vi "Penta Panes Demo.vi"() -> ()   [LabVIEW 2023]
doc: "Overview: Demonstrates the use of PentaPanes Class using a mockup of a GUI window. \nRequirements: Labview 2023 or compatible. \nInstructions: \n1. Run \"Penta Panes Demo.vi\" \n2. Play around with the GUI to see how it behaves. :)"
uses:
  Penta Panes.lvlibp/PanesColors.ctl
  <vilib>/Utility/miscctls.llb/LVBoundsTypeDef.ctl
  Penta Panes.lvlibp/ResizeBehaviourCluster.ctl
  Penta Panes.lvlibp/BordersCluster.ctl
  Penta Panes.lvlibp/1abvi3w/vi.lib/Utility/miscctls.llb/LVBoundsTypeDef.ctl
  Penta Panes.lvlibp/PanePosition.ctl
  <vilib>/Platform/browser.llb/Open URL in Default Browser (string).vi
  Penta Panes.lvlibp/5PanesGUI.lvclass
  Penta Panes.lvlibp
panel:
  out "Logo":picture[](array[picture])=[bytes[15730], bytes[15730], bytes[15730], bytes[15730], bytes[15730], bytes[15730], bytes[15730], bytes[15730], bytes[15730], bytes[15730], bytes[15730], bytes[15730], bytes[15730], bytes[15730], bytes[15730], bytes[15730], bytes[15730], bytes[15730], bytes[15730], bytes[15730], bytes[15730], bytes[15730], bytes[15730], bytes[15730], bytes[15730], bytes[15730], bytes[15730], bytes[15730], bytes[15730], bytes[15730], bytes[15730], bytes[15730], bytes[15730], bytes[15730], bytes[15730], bytes[15730], bytes[15730], bytes[15730], bytes[15730], bytes[15730], bytes[15730], bytes[15730], bytes[15730], bytes[15730], bytes[15730], bytes[15730], bytes[15730], bytes[15730], bytes[15730], bytes[15730], bytes[15730], bytes[15730]]
  out "Icons Values":bool[](array[boolean])
  out "IconNames":string[](array[string])
  out "Icons":picture[](array[picture])=[bytes[7230], bytes[7230], bytes[7230], bytes[7230], bytes[7230], bytes[7230], bytes[7230], bytes[7230], bytes[7230], bytes[7230], bytes[7230], bytes[7230], bytes[7230], bytes[7230], bytes[7230], bytes[7230], bytes[7230], bytes[7230], bytes[7230], bytes[7230], bytes[7230], bytes[7230], bytes[7230], bytes[7230], bytes[7230], bytes[7230], bytes[7230], bytes[7230], bytes[7230], bytes[7230], bytes[7230], bytes[7230], bytes[7230], bytes[7230], bytes[7230], bytes[7230], bytes[7230], bytes[7230], bytes[7230], bytes[7230], bytes[7230], bytes[7230], bytes[7230], bytes[7230], bytes[7230], bytes[7230], bytes[7230], bytes[7230], bytes[7230], bytes[7230], bytes[7230], bytes[7230]]
  in  "Options Tree":string[](tree)=["About"]
  in  "Options Tab":T1(tab)
  in  "Developed By\nLEAP CODE\nLinking hardware \nwith software\n\nYoni Cohen":string="yoncoh@gmail.com"
  in  "Icon set by":string="https://icons8.com"
  out "about picture":picture
  in  "Graphs Layout":T2(ring)=enum."3 Line graphs"
  in  "Right Pane View":u16(ring) items=["First", "Second", "Third"]
  in  "Top Pane Size":i32=75 caption="Top"
  in  "Right Pane Size":i32=156 caption="Right" max=4000
  in  "Left Pane Size":i32=113 caption="Left"
  in  "Bottom Pane Size":i32=100 caption="Bottom"
  in  "Colors":T3
  out "FP Bounds":T4
  out "App Path":path=path "E:/Work/5PanesWindow/5PanesDemo.vi"
  out "Eventloop Error":errorcluster
  out "Init Error":errorcluster
  out "Intensity Graph 2":dbl[][](graph)
  out "XY Graph 3":cluster{dbl[], dbl[]}[](graph)
  out "XY Graph 2":cluster{dbl[], dbl[]}[](graph)
  out "XY Graph":cluster{dbl[], dbl[]}[](graph)
  out "Intensity Graph":dbl[][](graph)
  in  "Third pane Tab":enum32{"Page 1", "Page 2"}(tab)
  in  "First pane Tab":enum32{"Page 1", "Page 2"}(tab)
  in  "Second pane Tab":enum32{"Page 1", "Page 2"}(tab)
  in  "Listbox":i32(listbox)=-1
  # "Overview: A mockup of a GUI window demonstrating the use of \nthe \"PentaPanes\" Class\nRequirements: LabVIEW 2023 or \ncompatible \nInstructions: Run this VI and play \naround with the GUI. \nopen and close panes by pressing the white splitters."
  # "Panes"
  # "Sizes"
  # "Debug Pane"
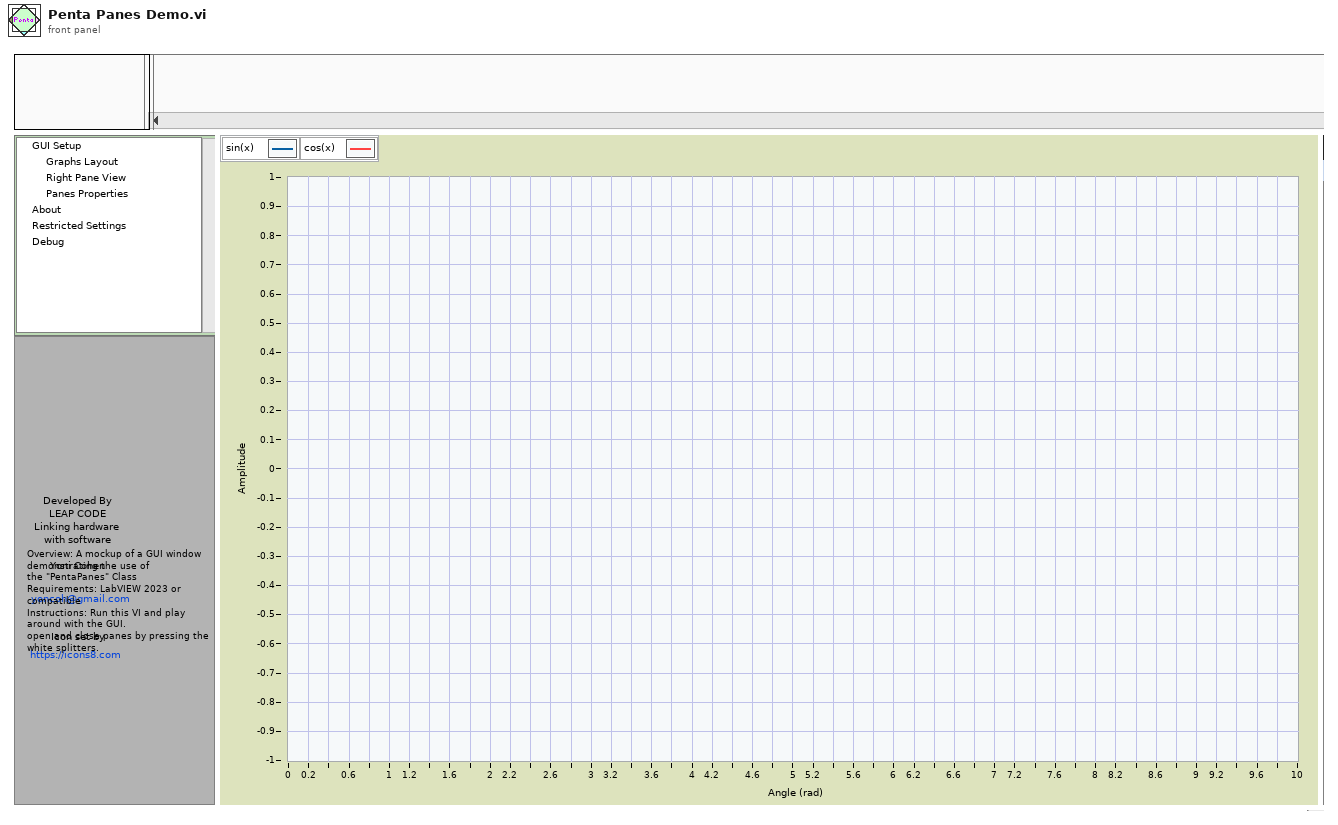
[diagram p1: front panel]
types:
  T1 = enum32{"About", "Graphs Layout", "Right Pane View", "Panes Colors", "Panes Properties", "Debug", "Restricted Settings"}
  T2 = enum16{"1 Line Graph", "1 Line + 2 Intensity", "3 Line graphs", "1 Intensity", "2 Intensity H", "2 Intensity V", "All"}
  T3 = typedef "Penta Panes.lvlibp/5PanesGUI.lvclass/PanesColors.ctl" = cluster{"Top Color":u32, "Left Color":u32, "Center Color":u32, "Right Color":u32, "Bottom Color":u32}
  T4 = typedef "LVBoundsTypeDef.ctl" = cluster{"Width":u32, "Height":u32}
  T5 = enum32{"Invalid", "Standard", "Closed", "Hidden", "Minimized", "Maximized"}
  T6 = enum16{"1 Line Graph", "1 Line + 2 Intensity", "3 Line graphs", "1 Intensity"}
  T7 = typedef "Penta Panes.lvlibp/5PanesGUI.lvclass/ResizeBehaviourCluster.ctl" = cluster{"Adjust":u16, "Borders":T8, "Borders in Percent?":bool, "Minimal":T9, "Invisible?":bool, "Force aspect ratio?":bool}
  T8 = typedef "Penta Panes.lvlibp/5PanesGUI.lvclass/BordersCluster.ctl" = cluster{"Left":i32, "Top":i32, "Right":i32, "Bottom":i32}
  T9 = typedef "Penta Panes.lvlibp/LVBoundsTypeDef.ctl" = cluster{"Width":u32, "Height":u32}
  T10 = typedef "LVRectTypeDef.ctl" = cluster{"Left":i16, "Top":i16, "Right":i16, "Bottom":i16}
  T11 = typedef "Penta Panes.lvlibp/5PanesGUI.lvclass/PanePosition.ctl" = u16
  T12 = typedef "LVPoint32TypeDef.ctl" = cluster{"Horizontal":i32, "Vertical":i32}
  T13 = typedef "LVRangeTypeDef.ctl" = cluster{"Minimum":dbl, "Maximum":dbl, "Increment":dbl, "Minor Increment":dbl, "Start":dbl}
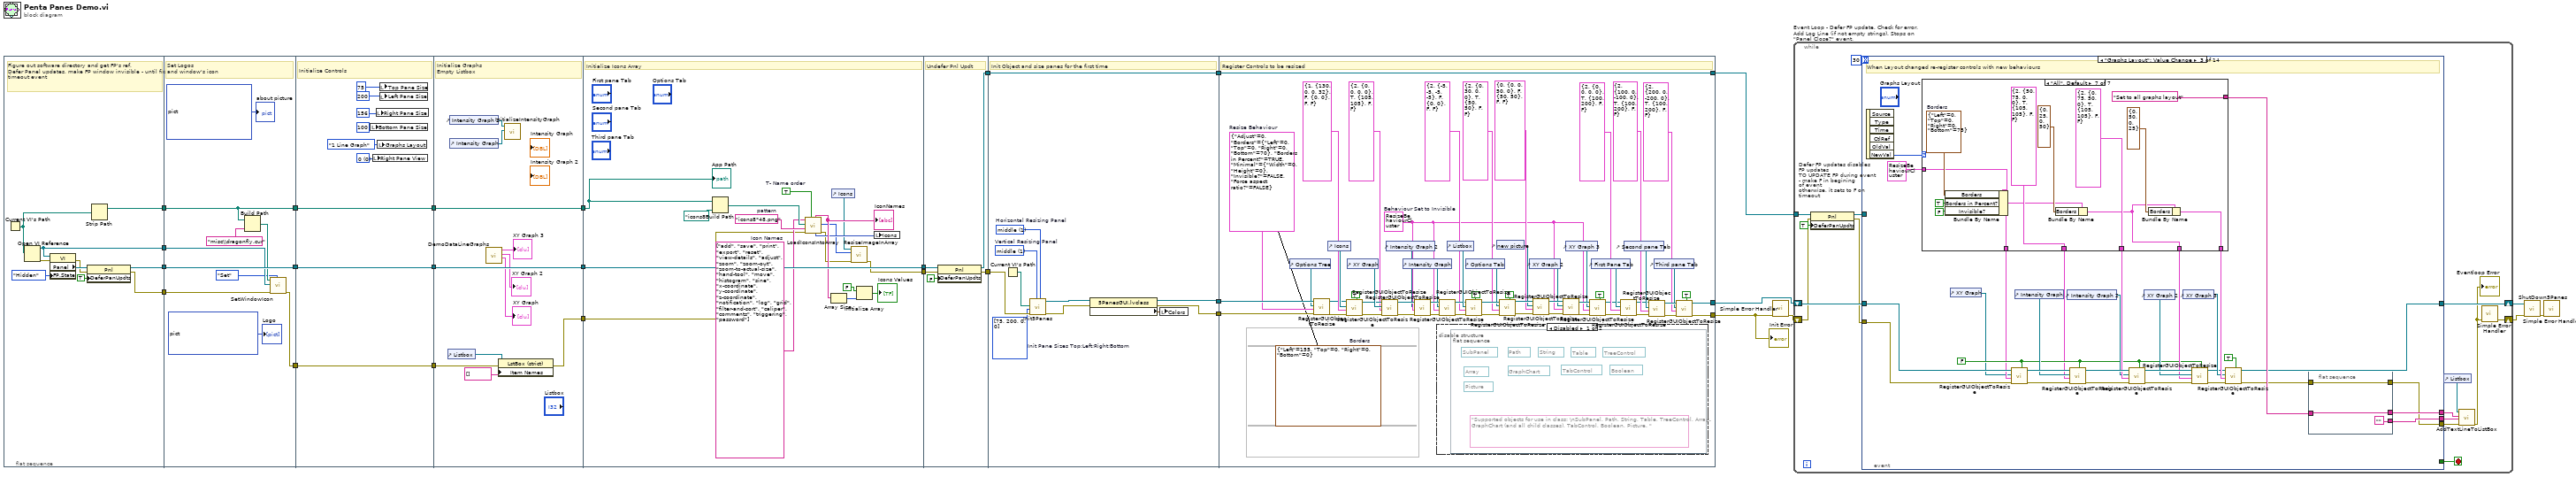
[diagram p0: block diagram]
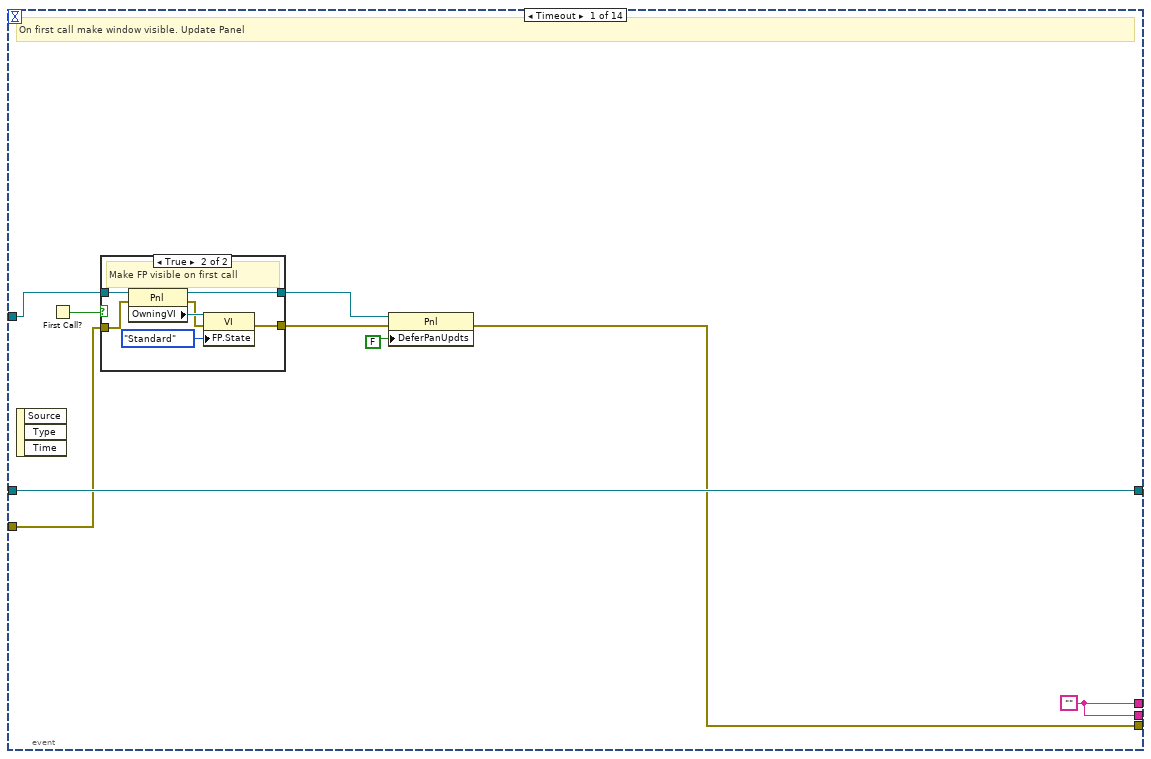
[diagram p3: hidden frame]
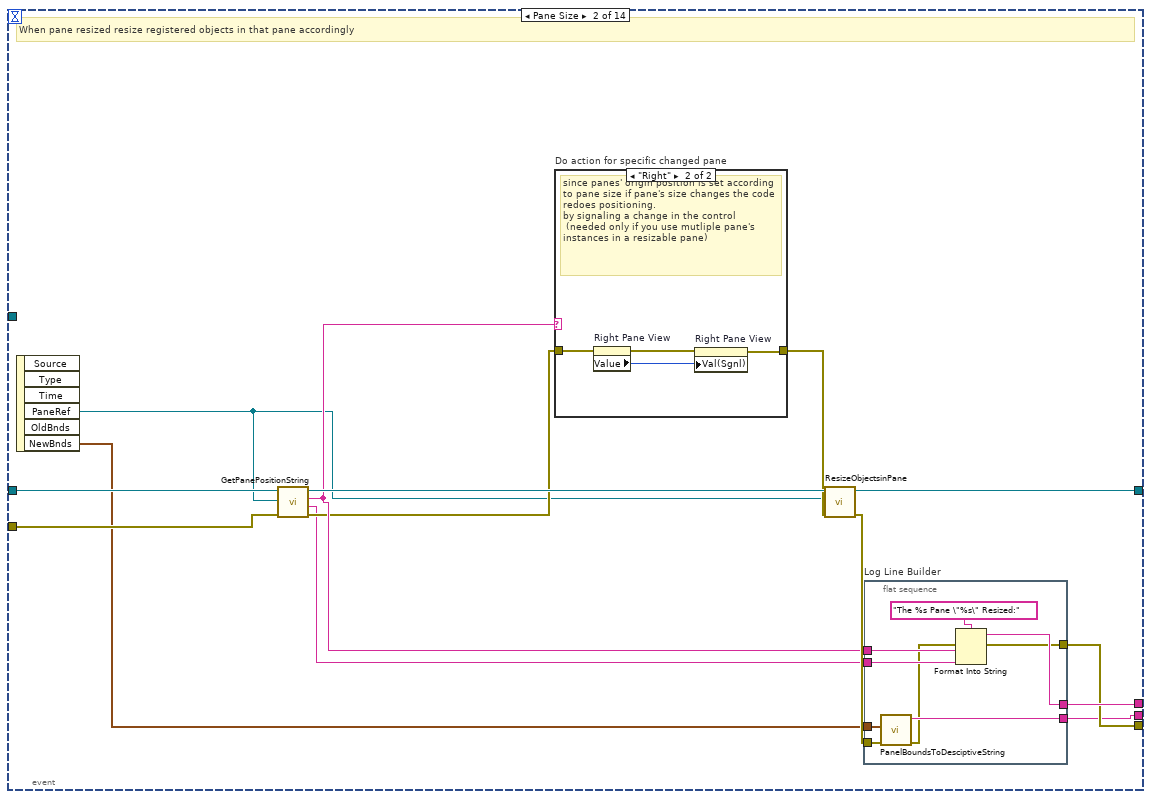
[diagram p5: hidden frame]
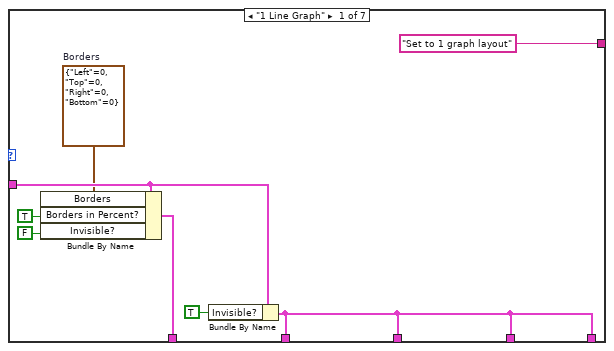
[diagram p7: hidden frame]
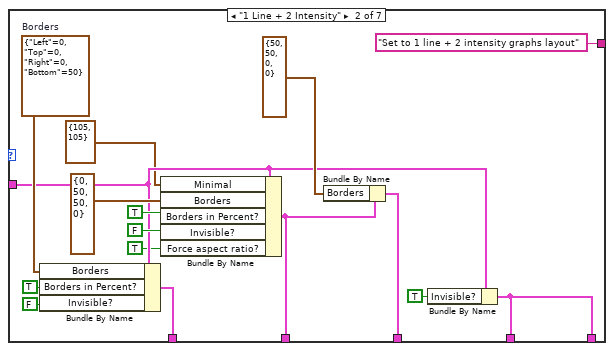
[diagram p8: hidden frame]
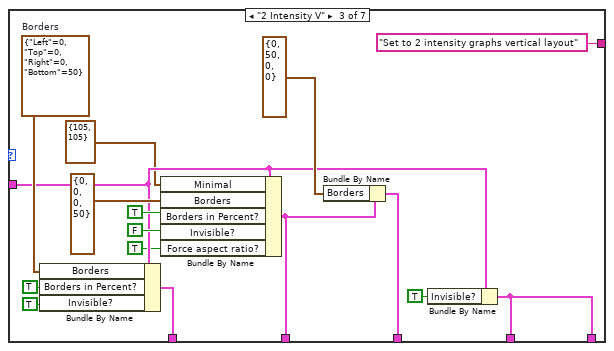
[diagram p9: hidden frame]
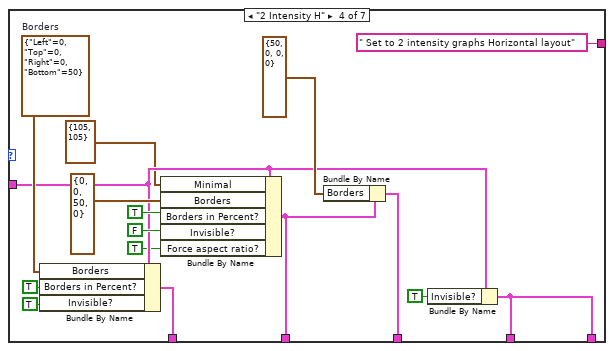
[diagram p10: hidden frame]
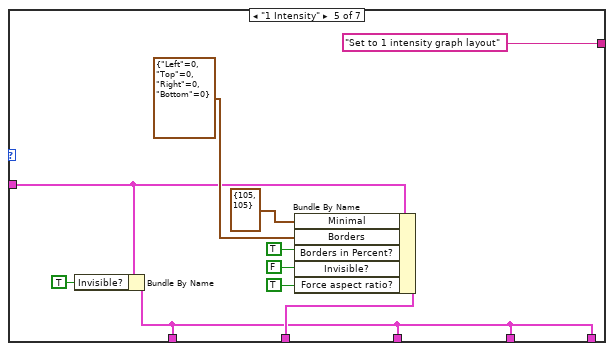
[diagram p11: hidden frame]
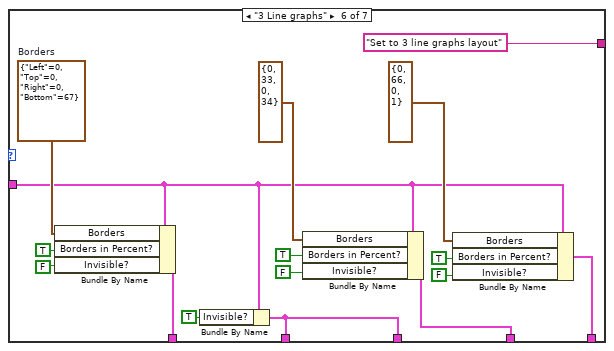
[diagram p12: hidden frame]
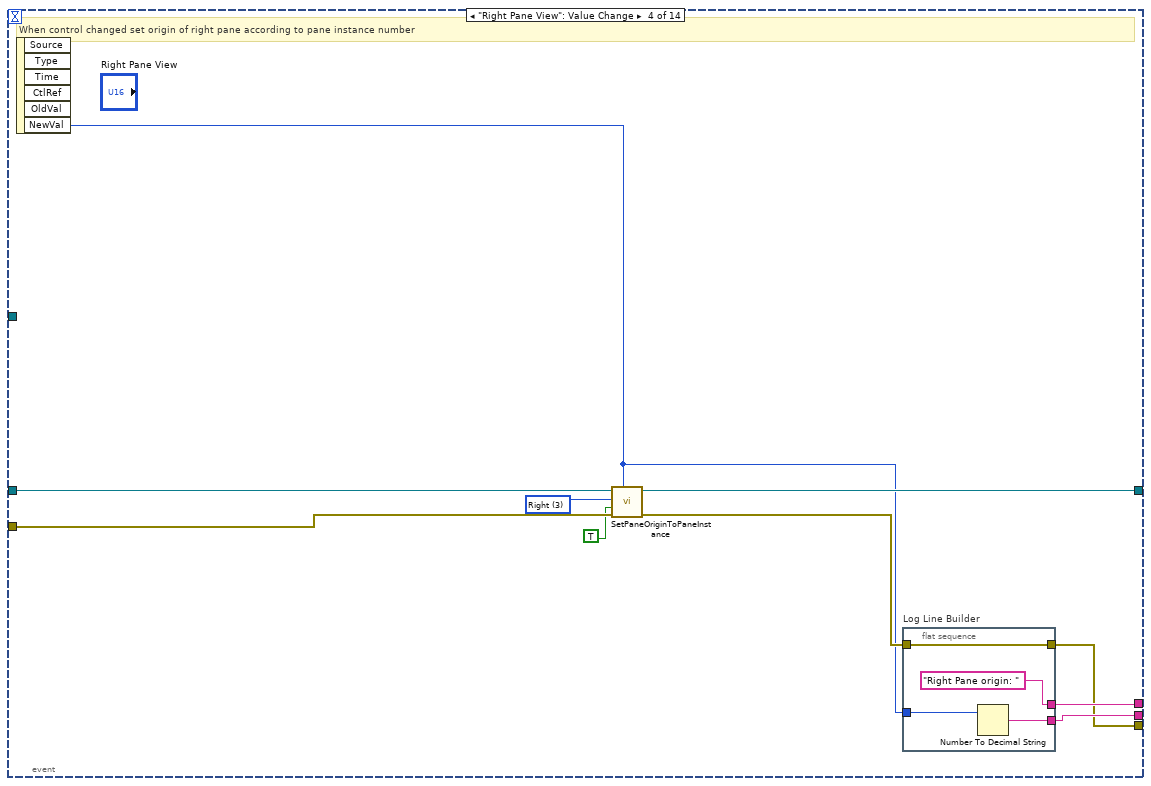
[diagram p13: hidden frame]
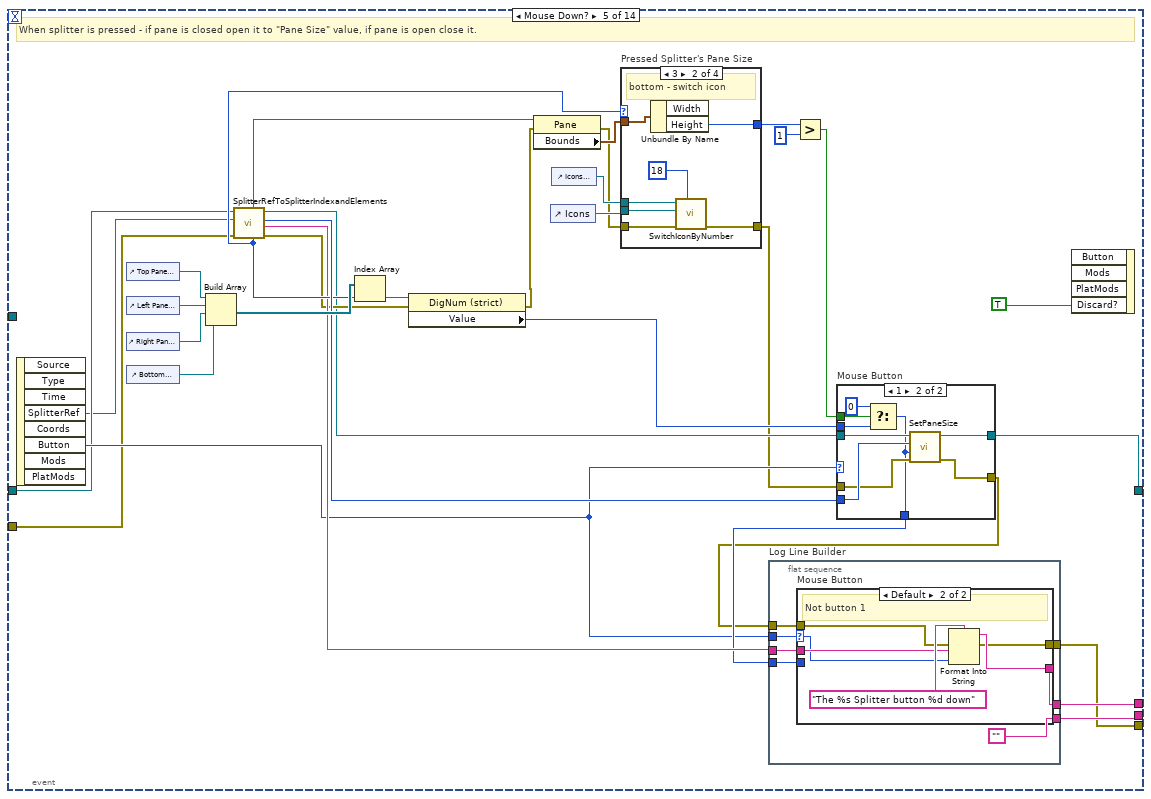
[diagram p14: hidden frame]
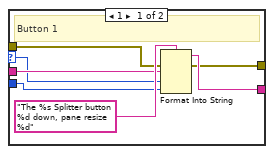
[diagram p15: hidden frame]
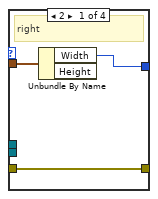
[diagram p16: hidden frame]
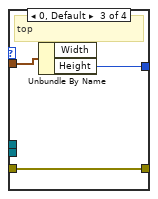
[diagram p17: hidden frame]
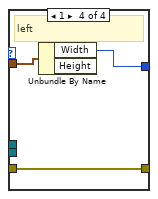
[diagram p18: hidden frame]
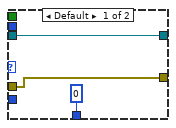
[diagram p19: hidden frame]
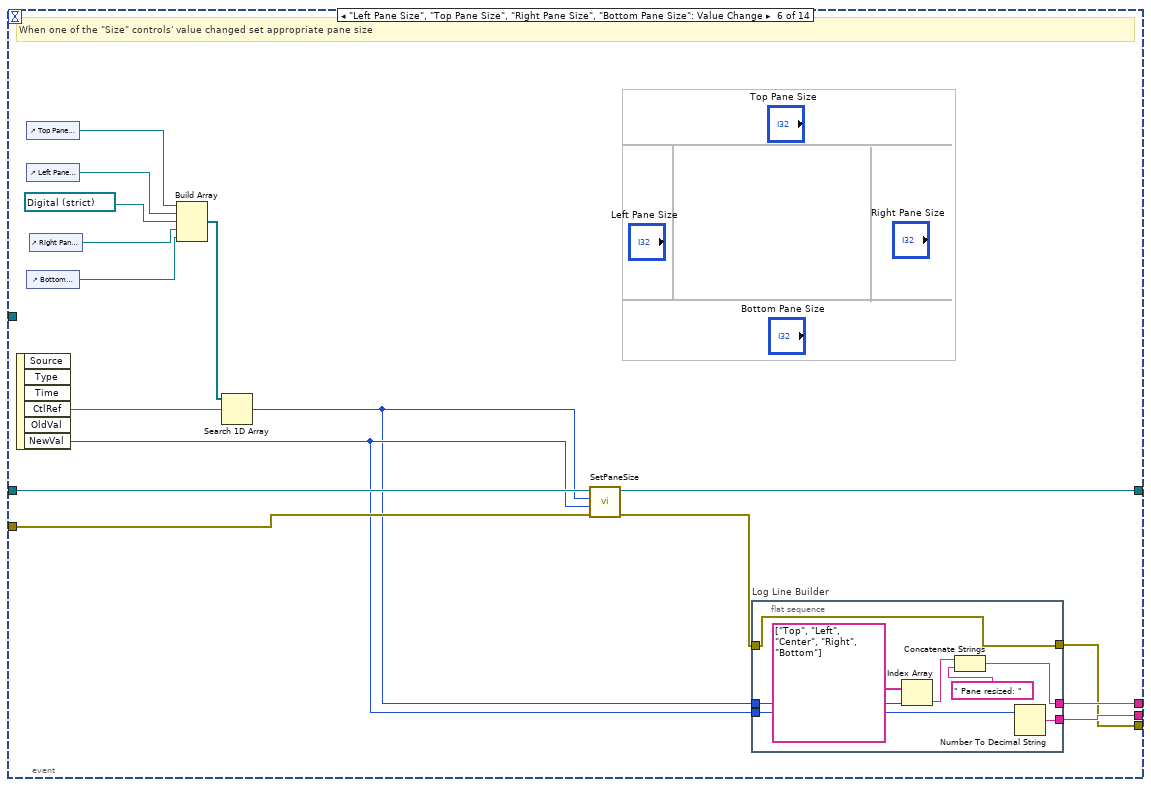
[diagram p20: hidden frame]
diagram:
  n1 = flat-sequence {
    tunnel: [w34] -> w12
    tunnel: [w32] -> w9
    tunnel: [w31] -> w8
    tunnel: [w29] -> w7
    tunnel: [w38] -> w13
    tunnel: w12 -> [w47]
    tunnel: [w47] -> w11
    tunnel: [w44] -> w10
    tunnel: w9 -> [w46]
    tunnel: w8 -> [w45]
    tunnel: w7 -> [w38]
    tunnel: w13 -> [w56]
    tunnel: [w56] -> w19
    tunnel: w11 -> [w55]
    tunnel: [w55] -> w17
    tunnel: [w48] -> w15
    tunnel: w10 -> [w48]
    tunnel: w19 -> [w67]
    tunnel: [w67] -> w18
    tunnel: w17 -> [w66]
    tunnel: [w66] -> w16
    tunnel: w15 -> [w59]
    tunnel: [w58] -> w14
    tunnel: [w84] -> w24
    tunnel: w18 -> [w74]
    tunnel: w16 -> [w84]
    tunnel: [w70] -> w21
    tunnel: w14 -> [w73]
    tunnel: w24 -> [w89]
    tunnel: w21 -> [w87]
    tunnel: [w86] -> w20
    tunnel: [w85] -> w2
    tunnel: [w91] -> w27
    tunnel: [w92] -> w26
    tunnel: w20 -> [w97]
    tunnel: [w90] -> w3
    tunnel: w2 -> [w90]
    tunnel: w27 -> [w123]
    tunnel: w26 -> [w127]
    tunnel: [w118] -> w5
    tunnel: [w117] -> w6
    tunnel: [w102] -> w1
    tunnel: w3 -> [w102]
    frame #0 {
      # "Figure out software directory and get FP's ref,\nDefer Panel updates, make FP window invisible - until first timeout event"
      n2 = Current VI's Path() -> (path=w30:path)
      n3 = Open VI Reference(vi path=w30) -> (vi reference=w31:refnum<vi>, error out=w36:errorcluster)  [unwired: 5 in]
      n4 = property on="Property Node" class="VI"(reference=w31, error in=w36, "FP.State"=T5."Hidden" ("Front Panel Window:State")) -> (error out=w33:errorcluster, "Panel"=w37:refnum<vi>)  [unwired: 1 out]
      n5 = property on="Property Node" class="Pnl"(reference=w37, error in=w33, "DeferPanUpdts"=TRUE ("Defer Panel Updates")) -> (reference out=w34:refnum<vi>, error out=w32:errorcluster)
      n6 = Strip Path(path=w30) -> (stripped path=w29:path)  [unwired: 1 out]
    }
    frame #1 {
      # "Set Logos \nand window's icon"
      n7 = Build Path(base path=w38, name or relative path="misc\\dragonfly.cur") -> (appended path=w43:path)
      n8 = call "SetWindowIcon.vi"("Action"=enum16{"Set", "Reset"}."Set", "error in (no error)"=w46, "VIRef (calling VI)"=w45, "ICO Icon"=w43) -> ("Error Out"=w44:errorcluster)  [unwired: 7 in]
      "Logo" <- picture[] [bytes[29955]] ("Logo")
      "about picture" <- picture bytes[70768] ("new picture")
    }
    frame #2 {
      w51 = u16 0 items=["0", "1", "2"] ("Right Pane Origin")
      # "Initialize Controls"
      n9 = local write "Bottom Pane Size"(100 ("Bottom Pane Size")) -> ()
      n10 = local write "Right Pane View"(w51) -> ()
      n11 = local write "Right Pane Size"(156 ("Right Pane Size")) -> ()
      n12 = local write "Graphs Layout"(T6."1 Line Graph" ("Graphs Layout")) -> ()
      n13 = local write "Top Pane Size"(75 ("Top Pane Size")) -> ()
      n14 = local write "Left Pane Size"(200 ("Top Pane Size")) -> ()
    }
    frame #3 {
      # "Initialize Graphs\nEmpty Listbox"
      n15 = control-ref of="Listbox"() -> (w57:refnum<vi>)
      n16 = control-ref of="Intensity Graph 2"() -> (w64:refnum<vi>)
      n17 = control-ref of="Intensity Graph"() -> (w65:refnum<vi>)
      n18 = call "DemoDataLineGraphs.vi"() -> (1:"XY Graph 3"=→"XY Graph":cluster{"X":dbl[], "Y":dbl[]}[], "XY Graph 2"=→"XY Graph 2":cluster{"X":dbl[], "Y":dbl[]}[], 3:"XY Graph 3"=→"XY Graph 3":cluster{"X":dbl[], "Y":dbl[]}[])  [unwired: 9 in]
      n19 = property on="Property Node" class="LstBox (strict)"(reference=w57, error in=w59, "Item Names"=string[] []) -> (error out=w58:errorcluster)  [unwired: 1 out]
      n20 = call "InitializeIntensityGraph.vi"("Intensity Graph 1 in"=w65, "IntensityGraph 2 in"=w64) -> ()  [unwired: 10 in]
    }
    frame #4 {
      w68 = TRUE  # T- Name order
      w76 = string[] ["add", "save", "print", "export", "reset", "view-details", "adjust", "zoom", "zoom-out", "zoom-to-actual-size", "hand-tool", "move", "histogram", "sine", "x-coordinate", "y-coordinate", "z-coordinate", "notification", "log", "grid", "filter-and-sort", "caliper", "comments", "triggering", "password"]  # Icon Names
      w77 = "icons8*48.png"  # pattern
      # "Initialize Icons Array"
      n21 = Build Path(base path=w74, name or relative path=path "icons8") -> (appended path=w78:path)
      n22 = call "LoadIconsIntoArray.vi"("T- Name order/F-File order"=w68, "error in"=w73, "Pattern"=w77, "Path to PNG files"=w78, "Name Order in"=w76) -> ("error out"=w71:errorcluster, "Icon Sizes"=w69:i32[], "Icons out"=w75:picture[], "Names out"=w83:string[])  [unwired: 2 in, 1 out]
      "IconNames" <- w83
      n23 = Array Size(array=w83) -> (size(s)=w81:i32)
      n24 = control-ref of="Icons"() -> (w72:refnum<vi>)
      n25 = call "ResizeImageInArray.vi"("error in (no error)"=w71, "Draw Area Width/Height"=w69, "Array in"=w72) -> ("error out"=w70:errorcluster)  [unwired: 8 in]
      n26 = Initialize Array(FALSE, w81) -> (→"Icons Values":bool[])
      n27 = local write "Icons"(w75) -> ()
      "App Path" <- w74
    }
    frame #5 {
      # "Undefer Pnl Updt"
      n28 = property on="Property Node" class="Pnl"(reference=w89, error in=w87, "DeferPanUpdts"=FALSE ("Defer Panel Updates")) -> (reference out=w85:refnum<vi>, error out=w86:errorcluster)
    }
    frame #6 {
      w93 = i32[] [75, 200, 0, 0]  # Init Pane Sizes Top;Left;Right;Bottom
      w98 = u16 1 items=["left", "middle", "right"]  # Horizontal Resizing Panel
      w99 = u16 1 items=["top", "middle", "bottom"]  # Vertical Resizing Panel
      # "Init Object and size panes for the first time"
      n29 = Current VI's Path() -> (path=w96:path)
      n30 = call "Init5Panes.vi"("Horizontal Resizing Pane"=w98, "Vertical Resizing Pane"=w99, "error in (no error)"=w97, "Pane Sizes Top;Left;Right;Bottom"=w93, "Path"=w96) -> ("error out"=w100:errorcluster, "5PanesGUI out"=w95:refnum<class "5PanesGUI.lvclass">)  [unwired: 4 in, 1 out]
      n31 = property on="Property Node" class="5PanesGUI.lvclass"(reference=w95, error in=w100) -> (reference out=w92:refnum<class "5PanesGUI.lvclass">, error out=w91:errorcluster, "Public Methods:Helpers:Panes Colors"=w94:T3)
      n32 = local write "Colors"(w94) -> ()
    }
    frame #7 {
      (unwired) T8 {"Left"=155, "Top"=0, "Right"=0, "Bottom"=0}  # Borders
      w133 = T7 {"Adjust"=2, "Borders"={"Left"=4000, "Top"=0, "Right"=0, "Bottom"=0}, "Borders in Percent?"=FALSE, "Minimal"={"Width"=0, "Height"=0}, "Invisible?"=TRUE, "Force aspect ratio?"=TRUE}  # Behaviour Set to Invisible
      w124 = T7 {"Adjust"=0, "Borders"={"Left"=0, "Top"=0, "Right"=0, "Bottom"=70}, "Borders in Percent?"=TRUE, "Minimal"={"Width"=0, "Height"=0}, "Invisible?"=FALSE, "Force aspect ratio?"=FALSE}  # Resize Behaviour
      # "Register Controls to be resized"
      n33 = control-ref of="Options Tree"() -> (w121:refnum<vi>)
      n34 = call-dynamic "RegisterGUIObjectToResize.vi"("error in (no error)"=w123, "Behaviour"=w124, "Any Control reference"=w121, "5PanesGUI in"=w127) -> ("error out"=w109:errorcluster, "5PanesGUI out"=w110:refnum<class "5PanesGUI.lvclass">)  [unwired: 4 in, 2 out]
      n35 = control-ref of="Icons"() -> (w126:refnum<vi>)
      n36 = call-dynamic "RegisterGUIObjectToResize.vi"("Resize Object?"=TRUE, "error in (no error)"=w109, "Behaviour"=T7 {"Adjust"=1, "Borders"={"Left"=130, "Top"=0, "Right"=0, "Bottom"=32}, "Borders in Percent?"=FALSE, "Minimal"={"Width"=0, "Height"=0}, "Invisible?"=FALSE, "Force aspect ratio?"=FALSE}, "Any Control reference"=w126, "5PanesGUI in"=w110) -> ("error out"=w144:errorcluster, "5PanesGUI out"=w143:refnum<class "5PanesGUI.lvclass">)  [unwired: 3 in, 2 out]
      n37 = control-ref of="XY Graph"() -> (w155:refnum<vi>)
      n38 = call-dynamic "RegisterGUIObjectToResize.vi"("error in (no error)"=w144, "Behaviour"=T7 {"Adjust"=2, "Borders"={"Left"=0, "Top"=0, "Right"=0, "Bottom"=0}, "Borders in Percent?"=TRUE, "Minimal"={"Width"=105, "Height"=105}, "Invisible?"=FALSE, "Force aspect ratio?"=FALSE} ("output cluster 2"), "Any Control reference"=w155, "5PanesGUI in"=w143) -> ("error out"=w146:errorcluster, "5PanesGUI out"=w151:refnum<class "5PanesGUI.lvclass">)  [unwired: 4 in, 2 out]
      n39 = control-ref of="Intensity Graph 2"() -> (w132:refnum<vi>)
      n40 = control-ref of="Intensity Graph"() -> (w148:refnum<vi>)
      n41 = call-dynamic "RegisterGUIObjectToResize.vi"("error in (no error)"=w146, "Behaviour"=w133, "Any Control reference"=w132, "5PanesGUI in"=w151) -> ("error out"=w147:errorcluster, "5PanesGUI out"=w150:refnum<class "5PanesGUI.lvclass">)  [unwired: 4 in, 2 out]
      n42 = disable-structure "Diagram Disable Structure" shown="Disabled" {
        frame Disabled {
          n43 = flat-sequence {
            frame #0 {
              (unwired) "Supported objects for use in class: \nSubPanel, Path, String, Table, TreeControl, Array, GraphChart (and all child classes), TabControl, Boolean, Picture. "
              (unwired) refnum<vi> refnum ("XY Graph")
              (unwired) refnum<vi> refnum ("XY Graph")
              (unwired) refnum<vi> refnum ("XY Graph")
              (unwired) refnum<vi> refnum ("XY Graph")
              (unwired) refnum<vi> refnum ("XY Graph")
              (unwired) refnum<vi> refnum ("XY Graph")
              (unwired) refnum<vi> refnum ("XY Graph")
              (unwired) refnum<vi> refnum ("XY Graph")
              (unwired) refnum<vi> refnum ("XY Graph")
              (unwired) refnum<vi> refnum ("XY Graph")
            }
          }
        }
        frame Enabled {
        }
      }
      n44 = call-dynamic "RegisterGUIObjectToResize.vi"("error in (no error)"=w147, "Behaviour"=w133, "Any Control reference"=w148, "5PanesGUI in"=w150) -> ("error out"=w145:errorcluster, "5PanesGUI out"=w149:refnum<class "5PanesGUI.lvclass">)  [unwired: 4 in, 2 out]
      n45 = control-ref of="Listbox"() -> (w154:refnum<vi>)
      n46 = control-ref of="Options Tab"() -> (w122:refnum<vi>)
      n47 = call-dynamic "RegisterGUIObjectToResize.vi"("Resize Object?"=TRUE, "error in (no error)"=w145, "Behaviour"=T7 {"Adjust"=2, "Borders"={"Left"=-5, "Top"=-5, "Right"=-5, "Bottom"=-5}, "Borders in Percent?"=FALSE, "Minimal"={"Width"=0, "Height"=0}, "Invisible?"=FALSE, "Force aspect ratio?"=FALSE} ("output cluster 5"), "Any Control reference"=w154, "5PanesGUI in"=w149) -> ("error out"=w156:errorcluster, "5PanesGUI out"=w157:refnum<class "5PanesGUI.lvclass">)  [unwired: 3 in, 2 out]
      n48 = control-ref of="new picture"() -> (w103:refnum<vi>)
      n49 = call-dynamic "RegisterGUIObjectToResize.vi"("Resize Object?"=TRUE, "error in (no error)"=w156, "Behaviour"=T7 {"Adjust"=2, "Borders"={"Left"=0, "Top"=30, "Right"=0, "Bottom"=0}, "Borders in Percent?"=TRUE, "Minimal"={"Width"=50, "Height"=50}, "Invisible?"=FALSE, "Force aspect ratio?"=FALSE} ("output cluster 6"), "Any Control reference"=w122, "5PanesGUI in"=w157) -> ("error out"=w152:errorcluster, "5PanesGUI out"=w153:refnum<class "5PanesGUI.lvclass">)  [unwired: 3 in, 2 out]
      n50 = control-ref of="XY Graph 2"() -> (w134:refnum<vi>)
      n51 = call-dynamic "RegisterGUIObjectToResize.vi"("error in (no error)"=w152, "Behaviour"=T7 {"Adjust"=0, "Borders"={"Left"=0, "Top"=0, "Right"=50, "Bottom"=0}, "Borders in Percent?"=FALSE, "Minimal"={"Width"=50, "Height"=50}, "Invisible?"=FALSE, "Force aspect ratio?"=FALSE} ("output cluster 7"), "Any Control reference"=w103, "5PanesGUI in"=w153) -> ("error out"=w135:errorcluster, "5PanesGUI out"=w138:refnum<class "5PanesGUI.lvclass">)  [unwired: 4 in, 2 out]
      n52 = call-dynamic "RegisterGUIObjectToResize.vi"("error in (no error)"=w135, "Behaviour"=w133, "Any Control reference"=w134, "5PanesGUI in"=w138) -> ("error out"=w136:errorcluster, "5PanesGUI out"=w137:refnum<class "5PanesGUI.lvclass">)  [unwired: 4 in, 2 out]
      n53 = control-ref of="XY Graph 3"() -> (w101:refnum<vi>)
      n54 = call-dynamic "RegisterGUIObjectToResize.vi"("Resize Object?"=TRUE, "error in (no error)"=w136, "Behaviour"=w133, "Any Control reference"=w101, "5PanesGUI in"=w137) -> ("error out"=w111:errorcluster, "5PanesGUI out"=w114:refnum<class "5PanesGUI.lvclass">)  [unwired: 3 in, 2 out]
      n55 = control-ref of="First Pane Tab"() -> (w128:refnum<vi>)
      n56 = call-dynamic "RegisterGUIObjectToResize.vi"("error in (no error)"=w111, "Behaviour"=T7 {"Adjust"=2, "Borders"={"Left"=0, "Top"=0, "Right"=0, "Bottom"=0}, "Borders in Percent?"=TRUE, "Minimal"={"Width"=100, "Height"=200}, "Invisible?"=FALSE, "Force aspect ratio?"=FALSE}, "Any Control reference"=w128, "5PanesGUI in"=w114) -> ("error out"=w112:errorcluster, "5PanesGUI out"=w113:refnum<class "5PanesGUI.lvclass">)  [unwired: 4 in, 2 out]
      n57 = control-ref of="Second pane Tab"() -> (w131:refnum<vi>)
      n58 = call-dynamic "RegisterGUIObjectToResize.vi"("error in (no error)"=w112, "Behaviour"=T7 {"Adjust"=2, "Borders"={"Left"=100, "Top"=0, "Right"=-100, "Bottom"=0}, "Borders in Percent?"=TRUE, "Minimal"={"Width"=100, "Height"=200}, "Invisible?"=FALSE, "Force aspect ratio?"=FALSE}, "Any Control reference"=w131, "5PanesGUI in"=w113) -> ("error out"=w119:errorcluster, "5PanesGUI out"=w120:refnum<class "5PanesGUI.lvclass">)  [unwired: 4 in, 2 out]
      n59 = control-ref of="Third pane Tab"() -> (w116:refnum<vi>)
      n60 = call-dynamic "RegisterGUIObjectToResize.vi"("Resize Object?"=TRUE, "error in (no error)"=w119, "Behaviour"=T7 {"Adjust"=2, "Borders"={"Left"=200, "Top"=0, "Right"=-200, "Bottom"=0}, "Borders in Percent?"=TRUE, "Minimal"={"Width"=100, "Height"=200}, "Invisible?"=FALSE, "Force aspect ratio?"=FALSE}, "Any Control reference"=w116, "5PanesGUI in"=w120) -> ("error out"=w118:errorcluster, "5PanesGUI out"=w117:refnum<class "5PanesGUI.lvclass">)  [unwired: 3 in, 2 out]
    }
  }
  n61 = call <vilib>:"Simple Error Handler.vi"("error in (no error)"=w5) -> ("error out"=w4:errorcluster)  [unwired: 4 in, 4 out]
  n62 = while "Event Loop - Defer FP update, Check for error. Add Log Line (if not empty strings). Stops on \"Panel Close?\" event." {
    shift-right: [w170] -> w23
    shift-left: w6 -> [w171]
    shift-right: [w158] -> w25
    shift-left: w4 -> [w165]
    tunnel: w1 -> [w162]
    stop <- w172 stop-if-true
    # "Defer FP updates disables \nFP updates \nTO UPDATE FP during event - make F in begining\nof event\notherwise, it sets to F on timeout"
    n63 = property class="Pnl"(reference=w162, error in=w165, "DeferPanUpdts"=TRUE ("Defer Panel Updates")) -> (reference out=w164:refnum<vi>, error out=w166:errorcluster)
    n64 = event shown="[2] \"Graphs Layout\": Value Change" {
      selector: _ -> [_ _ _ _ _ _ _ _ _ _ _ _ _ _]
      dyn-events: _ -> [_ _ _ _ _ _ _ _ _ _ _ _ _ _]
      timeout: 30 -> [_ _ _ _ _ _ _ _ _ _ _ _ _ _]
      tunnel: [_ _ _ _ _ _ _ _ _ TRUE _ _ _ _] -> w172
      tunnel: w171 -> [w181 w202 w245 w355 w369 w444 w472 w491 w613 w627 w641 w666 w677 w690]
      tunnel: w166 -> [w176 w200 w220 w354 w364 w452 w470 w480 w604 w626 w633 w664 w674 w685]
      tunnel: [w181 w203 w223 w350 w392 w453 w471 w492 w613 w627 w640 w665 w677 w690] -> w170
      tunnel: [w178 w197 w246 w351 w370 w454 w465 w493 w614 w626 w642 w660 w676 w688] -> w160
      tunnel: [w180 w196 w247 w352 w377 w455 w467 w498 w615 "" ("String") w643 w662 w673 w686] -> w161
      tunnel: [w180 w204 w248 w353 w376 w456 w468 w497 w616 "VI closed" ("String") w644 w659 w675 "Opening icon set creator website: " ("String")] -> w169
      tunnel: w164 -> [w173 _ _ _ _ _ _ w484 _ _ _ _ _ _]
      event Timeout {
        w180 = "" ("Empty String Constant")
        # "On first call make window visible. Update Panel"
        n65 = event-data() -> ()  [unwired: 1 in, 3 out]
        n66 = First Call?() -> (First Call?: T/F=w177:bool)
        n67 = case shown="True" w177 {
          tunnel: w173 -> [w182 w190]
          tunnel: w176 -> [w183 w187]
          tunnel: [w183 w185] -> w175
          tunnel: [w182 w184] -> w174
          frame False {
          }
          frame True {
            # "Make FP visible on first call"
            n68 = property on="Property Node" class="Pnl"(reference=w190, error in=w187) -> (reference out=w184:refnum<vi>, error out=w186:errorcluster, "OwningVI"=w189:refnum<vi>)
            n69 = property on="Property Node" class="VI"(reference=w189, error in=w186, "FP.State"=T5."Standard" ("Front Panel Window:State")) -> (error out=w185:errorcluster)  [unwired: 1 out]
          }
        }
        n70 = property on="Property Node" class="Pnl"(reference=w174, error in=w175, "DeferPanUpdts"=FALSE ("Defer Panel Updates")) -> (error out=w178:errorcluster)  [unwired: 1 out]
      }
      event Pane Size {
        # "When pane resized resize registered objects in that pane accordingly"
        n71 = event-data() -> ("PaneRef"=w191:refnum<vi>, "NewBnds"=w198:T10)  [unwired: 1 in, 4 out]
        n72 = call "GetPanePositionString.vi"("error in (no error)"=w200, "PaneRef"=w191, "5PanesGUI in"=w202) -> ("error out"=w194:errorcluster, "Label.Text"=w192:string, "Pos String"=w195:string, "5PanesGUI out"=w201:refnum<class "5PanesGUI.lvclass">)  [unwired: 5 in]
        n73 = case "Do action for specific changed pane" shown="\"Right\"" w195 {
          tunnel: w194 -> [w205 w208]
          tunnel: [w205 w206] -> w193
          frame Default {
            # "do nothing"
          }
          frame "Right" {
            # "since panes' origin position is set according to pane size if pane's size changes the code redoes positioning.\nby signaling a change in the control\n (needed only if you use mutliple pane's instances in a resizable pane)"
            n74 = property on="Right Pane View" class="Ring (strict)"(error in=w208) -> (error out=w207:errorcluster, "Value"=w209:u16)  [unwired: 1 in, 1 out]
            n75 = property on="Right Pane View" class="Ring (strict)"(error in=w207, "Val(Sgnl)"=w209) -> (error out=w206:errorcluster)  [unwired: 1 in, 1 out]
          }
        }
        n76 = call-dynamic "ResizeObjectsinPane.vi"("error in (no error)"=w193, "PaneRef"=w191, "5PanesGUI in"=w201) -> ("error out"=w199:errorcluster, "5PanesGUI out"=w203:refnum<class "5PanesGUI.lvclass">)  [unwired: 7 in]
        n77 = flat-sequence "Log Line Builder" {
          tunnel: [w214] -> w204
          tunnel: w199 -> [w218]
          tunnel: w198 -> [w217]
          tunnel: [w210] -> w197
          tunnel: [w216] -> w196
          tunnel: w195 -> [w213]
          tunnel: w192 -> [w212]
          frame #0 {
            n78 = call "PanelBoundsToDesciptiveString.vi"("error in (no error)"=w218, "Panel Bounds"=w217) -> ("error out"=w211:errorcluster, "String"=w216:string)  [unwired: 8 in]
            n79 = Format Into String(format string="The %s Pane \"%s\" Resized:", error in=w211, w213, w212) -> (resulting string=w214:string, error out=w210:errorcluster)  [unwired: 1 in]
          }
        }
      }
      event "Graphs Layout": Value Change {
        w228 = FALSE ("Resize Object?")
        # "When Layout changed re-register controls with new behaviours"
        n80 = event-data() -> ("NewVal"=w239:T2)  [unwired: 1 in, 5 out]
        n81 = case shown="\"All\", Default" w239 {
          tunnel: [w250 w257 w273 w289 w310 w315 T7 {"Adjust"=2, "Borders"={"Left"=50, "Top"=75, "Right"=0, "Bottom"=0}, "Borders in Percent?"=TRUE, "Minimal"={"Width"=105, "Height"=105}, "Invisible?"=FALSE, "Force aspect ratio?"=FALSE} ("output cluster")] -> w226
          tunnel: [w251 w269 w285 w301 w306 w327 w332] -> w227
          tunnel: ["Set to 1 graph layout" ("String") "Set to 1 line + 2 intensity graphs layout" ("String") "Set to 2 intensity graphs vertical layout" ("String") " Set to 2 intensity graphs Horizontal layout" ("String") "Set to 1 intensity graph layout" ("String") "Set to 3 line graphs layout" ("String") "Set to all graphs layout" ("String")] -> w236
          tunnel: T7 {"Adjust"=2, "Borders"={"Left"=0, "Top"=0, "Right"=0, "Bottom"=0}, "Borders in Percent?"=FALSE, "Minimal"={"Width"=100, "Height"=100}, "Invisible?"=FALSE, "Force aspect ratio?"=FALSE} ("Resize Behaviour") -> [w252 w262 w278 w294 w308 w317 w335]
          tunnel: [w250 w263 w279 w295 w306 w315 T7 {"Adjust"=2, "Borders"={"Left"=0, "Top"=75, "Right"=50, "Bottom"=0}, "Borders in Percent?"=TRUE, "Minimal"={"Width"=105, "Height"=105}, "Invisible?"=FALSE, "Force aspect ratio?"=FALSE} ("output cluster 2")] -> w235
          tunnel: [w250 w261 w277 w293 w306 w322 w331] -> w230
          tunnel: [w250 w261 w277 w293 w306 w321 w337] -> w233
          frame "1 Line Graph" {
            w249 = T8 {"Left"=0, "Top"=0, "Right"=0, "Bottom"=0}  # Borders
            n82 = Bundle By Name(cluster=w252, "Borders"=w249, "Borders in Percent?"=TRUE, "Invisible?"=FALSE) -> (w251:T7)
            n83 = Bundle By Name(cluster=w252, "Invisible?"=TRUE) -> (w250:T7)
          }
          frame "1 Line + 2 Intensity" {
            w271 = T8 {"Left"=0, "Top"=0, "Right"=0, "Bottom"=50}  # Borders
            n84 = Bundle By Name(cluster=w262, "Borders"=w271, "Borders in Percent?"=TRUE, "Invisible?"=FALSE) -> (w269:T7)
            n85 = Bundle By Name(cluster=w262, "Minimal"=T9 {"Width"=105, "Height"=105}, "Borders"=T8 {"Left"=0, "Top"=50, "Right"=50, "Bottom"=0}, "Borders in Percent?"=TRUE, "Invisible?"=FALSE, "Force aspect ratio?"=TRUE ("Force Aspect Ratio?")) -> (w257:T7)
            n86 = Bundle By Name(cluster=w257, "Borders"=T8 {"Left"=50, "Top"=50, "Right"=0, "Bottom"=0}) -> (w263:T7)
            n87 = Bundle By Name(cluster=w262, "Invisible?"=TRUE) -> (w261:T7)
          }
          frame "2 Intensity V" {
            w287 = T8 {"Left"=0, "Top"=0, "Right"=0, "Bottom"=50}  # Borders
            n88 = Bundle By Name(cluster=w278, "Borders"=w287, "Borders in Percent?"=TRUE, "Invisible?"=TRUE) -> (w285:T7)
            n89 = Bundle By Name(cluster=w278, "Minimal"=T9 {"Width"=105, "Height"=105}, "Borders"=T8 {"Left"=0, "Top"=0, "Right"=0, "Bottom"=50}, "Borders in Percent?"=TRUE, "Invisible?"=FALSE, "Force aspect ratio?"=TRUE ("Force Aspect Ratio?")) -> (w273:T7)
            n90 = Bundle By Name(cluster=w273, "Borders"=T8 {"Left"=0, "Top"=50, "Right"=0, "Bottom"=0}) -> (w279:T7)
            n91 = Bundle By Name(cluster=w278, "Invisible?"=TRUE) -> (w277:T7)
          }
          frame "2 Intensity H" {
            w303 = T8 {"Left"=0, "Top"=0, "Right"=0, "Bottom"=50}  # Borders
            n92 = Bundle By Name(cluster=w294, "Borders"=w303, "Borders in Percent?"=TRUE, "Invisible?"=TRUE) -> (w301:T7)
            n93 = Bundle By Name(cluster=w294, "Minimal"=T9 {"Width"=105, "Height"=105}, "Borders"=T8 {"Left"=0, "Top"=0, "Right"=50, "Bottom"=0}, "Borders in Percent?"=TRUE, "Invisible?"=FALSE, "Force aspect ratio?"=TRUE ("Force Aspect Ratio?")) -> (w289:T7)
            n94 = Bundle By Name(cluster=w289, "Borders"=T8 {"Left"=50, "Top"=0, "Right"=0, "Bottom"=0}) -> (w295:T7)
            n95 = Bundle By Name(cluster=w294, "Invisible?"=TRUE) -> (w293:T7)
          }
          frame "1 Intensity" {
            n96 = Bundle By Name(cluster=w308, "Invisible?"=TRUE) -> (w306:T7)
            n97 = Bundle By Name(cluster=w308, "Minimal"=T9 {"Width"=105, "Height"=105}, "Borders"=T8 {"Left"=0, "Top"=0, "Right"=0, "Bottom"=0}, "Borders in Percent?"=TRUE, "Invisible?"=FALSE, "Force aspect ratio?"=TRUE ("Force Aspect Ratio?")) -> (w310:T7)
          }
          frame "3 Line graphs" {
            w329 = T8 {"Left"=0, "Top"=0, "Right"=0, "Bottom"=67}  # Borders
            n98 = Bundle By Name(cluster=w317, "Borders"=w329, "Borders in Percent?"=TRUE, "Invisible?"=FALSE) -> (w327:T7)
            n99 = Bundle By Name(cluster=w317, "Invisible?"=TRUE) -> (w315:T7)
            n100 = Bundle By Name(cluster=w317, "Borders"=T8 {"Left"=0, "Top"=33, "Right"=0, "Bottom"=34}, "Borders in Percent?"=TRUE, "Invisible?"=FALSE) -> (w322:T7)
            n101 = Bundle By Name(cluster=w317, "Borders"=T8 {"Left"=0, "Top"=66, "Right"=0, "Bottom"=1}, "Borders in Percent?"=TRUE, "Invisible?"=FALSE) -> (w321:T7)
          }
          frame "All", Default {
            w341 = T8 {"Left"=0, "Top"=0, "Right"=0, "Bottom"=75}  # Borders
            n102 = Bundle By Name(cluster=w335, "Borders"=w341, "Borders in Percent?"=TRUE, "Invisible?"=FALSE) -> (w332:T7)
            n103 = Bundle By Name(cluster=w332, "Borders"=T8 {"Left"=0, "Top"=25, "Right"=0, "Bottom"=50}) -> (w331:T7)
            n104 = Bundle By Name(cluster=w331, "Borders"=T8 {"Left"=0, "Top"=50, "Right"=0, "Bottom"=25}) -> (w337:T7)
          }
        }
        n105 = control-ref of="XY Graph"() -> (w221:refnum<vi>)
        n106 = call-dynamic "RegisterGUIObjectToResize.vi"("Resize Object?"=w228, "error in (no error)"=w220, "Behaviour"=w227, "Any Control reference"=w221, "5PanesGUI in"=w245) -> ("error out"=w244:errorcluster, "5PanesGUI out"=w243:refnum<class "5PanesGUI.lvclass">)  [unwired: 3 in, 2 out]
        n107 = control-ref of="Intensity Graph"() -> (w242:refnum<vi>)
        n108 = control-ref of="Intensity Graph 2"() -> (w232:refnum<vi>)
        n109 = call-dynamic "RegisterGUIObjectToResize.vi"("Resize Object?"=w228, "error in (no error)"=w244, "Behaviour"=w226, "Any Control reference"=w242, "5PanesGUI in"=w243) -> ("error out"=w240:errorcluster, "5PanesGUI out"=w241:refnum<class "5PanesGUI.lvclass">)  [unwired: 3 in, 2 out]
        n110 = call-dynamic "RegisterGUIObjectToResize.vi"("Resize Object?"=w228, "error in (no error)"=w240, "Behaviour"=w235, "Any Control reference"=w232, "5PanesGUI in"=w241) -> ("error out"=w237:errorcluster, "5PanesGUI out"=w238:refnum<class "5PanesGUI.lvclass">)  [unwired: 3 in, 2 out]
        n111 = control-ref of="XY Graph 2"() -> (w231:refnum<vi>)
        n112 = control-ref of="XY Graph 3"() -> (w229:refnum<vi>)
        n113 = call-dynamic "RegisterGUIObjectToResize.vi"("Resize Object?"=w228, "error in (no error)"=w237, "Behaviour"=w230, "Any Control reference"=w231, "5PanesGUI in"=w238) -> ("error out"=w224:errorcluster, "5PanesGUI out"=w225:refnum<class "5PanesGUI.lvclass">)  [unwired: 3 in, 2 out]
        n114 = call-dynamic "RegisterGUIObjectToResize.vi"("Resize Object?"=TRUE, "error in (no error)"=w224, "Behaviour"=w233, "Any Control reference"=w229, "5PanesGUI in"=w225) -> ("error out"=w222:errorcluster, "5PanesGUI out"=w223:refnum<class "5PanesGUI.lvclass">)  [unwired: 3 in, 2 out]
        n115 = flat-sequence {
          tunnel: [w343] -> w248
          tunnel: ["" ("Empty String Constant")] -> w247
          tunnel: w222 -> [w345]
          tunnel: [w345] -> w246
          tunnel: w236 -> [w343]
          frame #0 {
          }
        }
      }
      event "Right Pane View": Value Change {
        w348 = u16 3 items=["Top", "Left", "Center", "Right", "Bottom"] ("Pane")
        # "When control changed set origin of right pane according to pane instance number"
        n116 = event-data() -> ("NewVal"=w347:u16)  [unwired: 1 in, 5 out]
        n117 = call "SetPaneOriginToPaneInstance.vi"("Pane number"=w347, "error in (no error)"=w354, "Panes Origin differ by - X(T) or Y(F)"=TRUE, "Pane"=w348, "5PanesGUI in"=w355) -> ("error out"=w349:errorcluster, "5PanesGUI out"=w350:refnum<class "5PanesGUI.lvclass">)  [unwired: 5 in]
        n118 = flat-sequence "Log Line Builder" {
          tunnel: w347 -> [w359]
          tunnel: ["Right Pane origin: " ("String")] -> w353
          tunnel: [w357] -> w352
          tunnel: w349 -> [w356]
          tunnel: [w356] -> w351
          frame #0 {
            n119 = Number To Decimal String(number=w359) -> (decimal integer string=w357:string)  [unwired: 1 in]
          }
        }
      }
      event Mouse Down? {
        # "When splitter is pressed - if pane is closed open it to \"Pane Size\" value, if pane is open close it."
        n120 = event-data() -> ("SplitterRef"=w366:refnum<vi>, "Button"=w372:u16)  [unwired: 1 in, 6 out]
        n121 = control-ref of="Top Pane Size"() -> (w391:refnum<vi>)
        n122 = control-ref of="Left Pane Size"() -> (w390:refnum<vi>)
        n123 = control-ref of="Right Pane Size"() -> (w389:refnum<vi>)
        n124 = control-ref of="Bottom Pane Size"() -> (w388:refnum<vi>)
        n125 = Build Array(w391, w390, w389, w388) -> (w387:refnum<vi>[])
        n126 = call "SplitterRefToSplitterIndexandElements.vi"("error in (no error)"=w364, "SplitterRef"=w366, "5PanesGUI in"=w369) -> ("error out"=w368:errorcluster, "Splitter String"=w374:string, "Splitter Pane Pos"=w383:T11, "5PanesGUI out"=w367:refnum<class "5PanesGUI.lvclass">, "Pressed Splitter Index Out"=w375:i32, "Pane Ref out"=w380:refnum<vi>)  [unwired: 3 in]
        n127 = Index Array(array=w387, index=w375) -> (element=w365:refnum<vi>)
        n128 = property on="Property Node" class="DigNum (strict)"(reference=w365, error in=w368) -> (error out=w378:errorcluster, "Value"=w386:i32)  [unwired: 1 out]
        n129 = property on="Property Node" class="Pane"(reference=w380, error in=w378) -> (error out=w361:errorcluster, "Bounds"=w384:T4)  [unwired: 1 out]
        n130 = control-ref of="Icons"() -> (w363:refnum<vi>)
        n131 = control-ref of="Icons Values"() -> (w362:refnum<vi>)
        n132 = case "Pressed Splitter's Pane Size" shown="3" w375 {
          tunnel: w384 -> [w415 w422 w425 w428]
          tunnel: [w414 w421 w424 w427] -> w382
          tunnel: w363 -> [_ w419 _ _]
          tunnel: w362 -> [_ w418 _ _]
          tunnel: w361 -> [w413 w417 w423 w426]
          tunnel: [w413 w416 w423 w426] -> w360
          frame 2 {
            # "right"
            n133 = Unbundle By Name(w415) -> ("Width"=w414:u32)  [unwired: 1 out]
          }
          frame 3 {
            # "bottom - switch icon"
            n134 = Unbundle By Name(w422) -> ("Height"=w421:u32)  [unwired: 1 out]
            n135 = call "SwitchIconByNumber.vi"("Index"=u32 18, "error in (no error)"=w417, "Icon Array Ref"=w419, "Switch Values ref"=w418) -> ("error out"=w416:errorcluster)  [unwired: 4 in, 3 out]
          }
          frame 0, Default {
            # "top"
            n136 = Unbundle By Name(w425) -> ("Height"=w424:u32)  [unwired: 1 out]
          }
          frame 1 {
            # "left"
            n137 = Unbundle By Name(w428) -> ("Width"=w427:u32)  [unwired: 1 out]
          }
        }
        n138 = flat-sequence "Log Line Builder" {
          tunnel: [w399] -> w376
          tunnel: [w397] -> w370
          tunnel: ["" ("String")] -> w377
          tunnel: w374 -> [w398]
          tunnel: w373 -> [w396]
          tunnel: w372 -> [w394]
          tunnel: w371 -> [w393]
          frame #0 {
            n139 = case "Mouse Button" shown="Default" w394 {
              selector: w394 -> [w401 w407]
              tunnel: [w405 w411] -> w399
              tunnel: w398 -> [w404 w410]
              tunnel: [w403 w409] -> w397
              tunnel: w396 -> [w402 _]
              tunnel: w393 -> [w400 w408]
              frame 1 {
                # "Button 1"
                n140 = Format Into String(format string="The %s Splitter button %d down, pane resize %d", error in=w400, w404, w401, w402) -> (resulting string=w405:string, error out=w403:errorcluster)  [unwired: 1 in]
              }
              frame Default {
                # "Not button 1"
                n141 = Format Into String(format string="The %s Splitter button %d down", error in=w408, w410, w407) -> (resulting string=w411:string, error out=w409:errorcluster)  [unwired: 1 in]
              }
            }
          }
        }
        n142 = Greater?(x=w382, y=u32 1) -> (0:w379:bool)
        n143 = case "Mouse Button" shown="1" w372 {
          tunnel: w367 -> [w431 w440]
          tunnel: [w431 w439] -> w392
          tunnel: w383 -> [_ w438]
          tunnel: w386 -> [_ w433]
          tunnel: w360 -> [w430 w436]
          tunnel: [w430 w437] -> w371
          tunnel: w379 -> [_ w435]
          tunnel: [0 ("Value") w432] -> w373
          frame Default {
          }
          frame 1 {
            n144 = Select(t=i16 0, s=w435, f=w433) -> (s? t:f=w432:i32)
            n145 = call "SetPaneSize.vi"("error in (no error)"=w436, "Pane Size"=w432, "Pane Position"=w438, "5PanesGUI in"=w440) -> ("error out"=w437:errorcluster, "5PanesGUI out"=w439:refnum<class "5PanesGUI.lvclass">)  [unwired: 6 in]
          }
        }
        n146 = event-data ("Event Filter Node")("Discard?"=TRUE) -> ()  [unwired: 4 in, 1 out]
      }
      event "Left Pane Size", "Top Pane Size", "Right Pane Size", "Bottom Pane Size": Value Change {
        # "When one of the \"Size\" controls' value changed set appropriate pane size"
        n147 = event-data() -> ("CtlRef"=w445:refnum<vi>, "NewVal"=w443:i32)  [unwired: 1 in, 4 out]
        n148 = control-ref of="Top Pane Size"() -> (w451:refnum<vi>)
        n149 = control-ref of="Left Pane Size"() -> (w450:refnum<vi>)
        n150 = control-ref of="Bottom Pane Size"() -> (w447:refnum<vi>)
        n151 = control-ref of="Right Pane Size"() -> (w448:refnum<vi>)
        n152 = Build Array(w451, w450, refnum<vi> refnum ("element"), w448, w447) -> (w446:refnum<vi>[])
        n153 = Search 1D Array(1D array=w446, element=w445) -> (index of element=w441:i32)  [unwired: 1 in]
        n154 = call "SetPaneSize.vi"("error in (no error)"=w452, "Pane Size"=w443, "Pane Position"=w441, "5PanesGUI in"=w444) -> ("error out"=w442:errorcluster, "5PanesGUI out"=w453:refnum<class "5PanesGUI.lvclass">)  [unwired: 6 in]
        n155 = flat-sequence "Log Line Builder" {
          tunnel: w443 -> [w457]
          tunnel: [w462] -> w456
          tunnel: [w464] -> w455
          tunnel: [w460] -> w454
          tunnel: w442 -> [w460]
          tunnel: w441 -> [w458]
          frame #0 {
            n156 = Index Array(array=string[] ["Top", "Left", "Center", "Right", "Bottom"], index=w458) -> (element=w461:string)
            n157 = Concatenate Strings(w461, " Pane resized: " ("String")) -> (w462:string)
            n158 = Number To Decimal String(number=w457) -> (decimal integer string=w464:string)  [unwired: 1 in]
          }
        }
      }
      event Value Change {
        # "When Pane Colors Change - Set to new pane colors"
        n159 = event-data() -> ("CtlRef"=w473:refnum<vi>, "NewVal"=w469:T3)  [unwired: 1 in, 4 out]
        n160 = call-dynamic "SetColors.vi"("error in (no error)"=w470, "Colors"=w469, "5PanesGUI in"=w472) -> ("error out"=w466:errorcluster, "5PanesGUI out"=w471:refnum<class "5PanesGUI.lvclass">)  [unwired: 7 in]
        n161 = flat-sequence "Log Line Builder" {
          tunnel: w473 -> [w478]
          tunnel: ["Panes colors set to: " ("String")] -> w468
          tunnel: [w476] -> w467
          tunnel: w466 -> [w475]
          tunnel: [w474] -> w465
          frame #0 {
            n162 = call "ClusterToDescriptiveString.vi"("error in"=w475, "Cluster In"=w478) -> ("error out"=w474:errorcluster, "String"=w476:string)  [unwired: 8 in]
          }
        }
      }
      event "Icons": Mouse Down? {
        # "When mouse click on icons array - Do \"Action for specific icon\""
        n163 = event-data() -> ("CtlRef"=w496:refnum<vi>, "Coords"=w495:T12, "Button"=w488:u16)  [unwired: 1 in, 5 out]
        n164 = control-ref of="IconNames"() -> (w490:refnum<vi>)
        n165 = control-ref of="Icons Values"() -> (w487:refnum<vi>)
        n166 = call "GetArrayIndexFromCoordinate.vi"("error in (no error)"=w480, "Coords in"=w495, "Array in"=w496) -> ("error out"=w479:errorcluster, "in element? (1D arrays only)"=w481:bool, "Element Indexes"=w483:cluster{"Horizontal":u32, "Vertical":u32}, "Array out"=w494:refnum<vi>)  [unwired: 3 in, 2 out]
        n167 = property on="Property Node" class="Pnl"(reference=w484, error in=w479, "DeferPanUpdts"=FALSE ("Defer Panel Updates")) -> (error out=w486:errorcluster)  [unwired: 1 out]
        n168 = Unbundle By Name(w483) -> ("Horizontal"=w482:u32)
        n169 = case shown="True" w481 {
          tunnel: [w503 w527] -> w498
          tunnel: [w503 w526] -> w497
          tunnel: w494 -> [_ w511]
          tunnel: w482 -> [_ w510]
          tunnel: w486 -> [w502 w522]
          tunnel: [w502 w514] -> w493
          tunnel: w491 -> [w501 w521]
          tunnel: [w501 w520] -> w492
          tunnel: w490 -> [_ w519]
          tunnel: [w500 TRUE ("Discard?")] -> w489
          tunnel: w488 -> [w499 _]
          tunnel: w487 -> [_ w512]
          frame False {
            w503 = "" ("Empty String Constant")
            # "not in element"
            n170 = case "Mouse button" shown="1" w499 {
              tunnel: [TRUE ("Discard?") TRUE ("Discard?") FALSE ("Discard?")] -> w500
              frame 0 {
              }
              frame Default {
              }
              frame 1 {
              }
            }
          }
          frame True {
            # "in element"
            n171 = property on="Property Node" class="Arr (strict)"(reference=w519, error in=w522) -> (error out=w517:errorcluster, "Value"=w525:string[])  [unwired: 1 out]
            n172 = call "SwitchIconByNumber.vi"("Index"=w510, "error in (no error)"=w517, "Icon Array Ref"=w511, "Switch Values ref"=w512) -> ("error out"=w516:errorcluster, "Val out"=w507:bool, "Icon Array ref out"=w508:refnum<vi>, "Switch Values ref out"=w509:refnum<vi>)  [unwired: 4 in]
            n173 = Index Array(array=w525, index=w510) -> (element=w524:string)
            n174 = case "Action for specific icon" shown="\"log\"" w524 {
              selector: w524 -> [w554 w569 w583 w592]
              tunnel: [w554 w569 w583 w592] -> w523
              tunnel: w516 -> [w551 w561 w576 w596]
              tunnel: [w551 w563 w581 w595] -> w515
              tunnel: w521 -> [w553 w555 w582 w594]
              tunnel: [w553 w564 w580 w593] -> w520
              tunnel: [w552 w568 w579 w591] -> w513
              tunnel: w507 -> [_ _ w574 w590]
              frame "Latch button name", Default {
                w552 = FALSE  # Switch(T)/Latch(F)
                (unwired) TRUE
                # "Duplicate this case for \"latch\" icon action"
                n175 = Wait (ms)(milliseconds to wait=u32 100) -> ()  [unwired: 1 out]
              }
              frame "zoom-to-actual-size" {
                w568 = FALSE  # Switch(T)/Latch(F)
                (unwired) TRUE
                # "Autoscale all graphs and resize objects in graph's pane (latch)"
                n176 = control-ref of="Intensity Graph"() -> (w557:refnum<vi>)
                n177 = control-ref of="Intensity Graph 2"() -> (w556:refnum<vi>)
                n178 = control-ref of="XY Graph"() -> (w559:refnum<vi>)
                n179 = control-ref of="XY Graph 2"() -> (w567:refnum<vi>)
                n180 = control-ref of="XY Graph 3"() -> (w566:refnum<vi>)
                n181 = Build Array(w559, w567, w566, w557, w556) -> (w565:refnum<vi>[])
                n182 = for {
                  tunnel: w565 -> [w573] mode=indexing
                  shift-right: [w570] -> w558
                  shift-left: w561 -> [w571]
                  w572 = u8 1 ("X Scale.Scale Fit")
                  n183 = property on="Property Node" class="GrphChrt"(reference=w573, error in=w571, "XScale.ScaleFit"=w572, "YScale.ScaleFit"=w572) -> (error out=w570:errorcluster)  [unwired: 1 out]
                }
                n184 = property on="Property Node" class="IntGraph (strict)"(reference=w556, error in=w558) -> (error out=w560:errorcluster, "OwningPane"=w562:refnum<vi>)  [unwired: 1 out]
                n185 = call-dynamic "ResizeObjectsinPane.vi"("error in (no error)"=w560, "PaneRef"=w562, "5PanesGUI in"=w555) -> ("error out"=w563:errorcluster, "5PanesGUI out"=w564:refnum<class "5PanesGUI.lvclass">)  [unwired: 7 in]
              }
              frame "log" {
                w577 = T11 4 items=["Top", "Left", "Center", "Right", "Bottom"] ("Pane Position")
                w579 = TRUE  # Switch(T)/Latch(F)
                # "open/close bottom (log) pane (switch)"
                n186 = case "Switch new Value" shown="True" w574 {
                  tunnel: [0 ("t") w588] -> w578
                  tunnel: w576 -> [w584 w587]
                  tunnel: [w584 w586] -> w575
                  frame False {
                    # "Close Bottom Pane"
                  }
                  frame True {
                    # "Show Bottom Pane"
                    n187 = control-ref of="Bottom Pane Size"() -> (w589:refnum<vi>)
                    n188 = property on="Property Node" class="DigNum (strict)"(reference=w589, error in=w587) -> (error out=w586:errorcluster, "Value"=w588:i32)  [unwired: 1 out]
                  }
                }
                n189 = call "SetPaneSize.vi"("error in (no error)"=w575, "Pane Size"=w578, "Pane Position"=w577, "5PanesGUI in"=w582) -> ("error out"=w581:errorcluster, "5PanesGUI out"=w580:refnum<class "5PanesGUI.lvclass">)  [unwired: 6 in]
              }
              frame "Switch button name" {
                w591 = TRUE  # Switch(T)/Latch(F)
                # "Duplicate this case for new \"switch\" icon actions"
                n190 = case "Switch new Value" shown="True" w590 {
                  tunnel: w596 -> [w598 w600]
                  tunnel: [w598 w600] -> w595
                  tunnel: w594 -> [w597 w599]
                  tunnel: [w597 w599] -> w593
                  tunnel: w592 -> [_ _]
                  frame False {
                    # "New Button Value - False"
                  }
                  frame True {
                    # "New Button Value - True"
                  }
                }
              }
            }
            n191 = flat-sequence "Log Line Builder" {
              tunnel: ["" ("Empty String Constant")] -> w527
              tunnel: w510 -> [w546]
              tunnel: [w547] -> w526
              tunnel: w523 -> [w543]
              tunnel: w513 -> [w542]
              tunnel: w507 -> [w541]
              frame #0 {
                n192 = Select(t="On" ("string"), s=w541, f="Off" ("string")) -> (s? t:f=w537:string)
                n193 = Number To Decimal String(number=w546) -> (decimal integer string=w545:string)  [unwired: 1 in]
                n194 = Concatenate Strings(" switched " ("string"), w537) -> (w536:string)
                n195 = Select(t=w536, s=w542, f=" pressed " ("string")) -> (s? t:f=w539:string)
                n196 = Concatenate Strings("Icon #" ("string"), w545, " " ("string"), w543, w539) -> (w547:string)
              }
            }
            n197 = case shown="False" w513 {
              tunnel: w515 -> [w532 w533]
              tunnel: [w531 w533] -> w514
              tunnel: w510 -> [w530 _]
              tunnel: w509 -> [w529 _]
              tunnel: w508 -> [w528 _]
              frame False {
                # "if Latch switch back off"
                n198 = call "SwitchIconByNumber.vi"("Index"=w530, "error in (no error)"=w532, "Icon Array Ref"=w528, "Switch Values ref"=w529) -> ("error out"=w531:errorcluster)  [unwired: 4 in, 3 out]
              }
              frame True {
              }
            }
          }
        }
        n199 = event-data ("Event Filter Node")("Discard?"=w489) -> ()  [unwired: 4 in, 1 out]
      }
      event "Options Tree": Value Change {
        # "When Tree Control changes value change to the tab page with the same name"
        n200 = event-data() -> ("NewVal"=w606:string[])  [unwired: 1 in, 5 out]
        n201 = Index Array(array=w606) -> (element=w605:string)  [unwired: 1 in]
        n202 = control-ref of="Options Tab"() -> (w612:refnum<vi>)
        n203 = property on="Property Node" class="TabCtl (strict)"(reference=w612, error in=w604) -> (reference out=w608:refnum<vi>, error out=w603:errorcluster, "Pages"=w611:refnum<vi>[])
        n204 = for {
          tunnel: w611 -> [w622] mode=indexing
          tunnel: w605 -> [w620]
          tunnel: [w619] -> w609 mode=indexing
          shift-right: [w617] -> w602
          shift-left: w603 -> [w618]
          n205 = property on="Property Node" class="Page"(reference=w622, error in=w618) -> (error out=w617:errorcluster, "PageLabel"=w621:string)  [unwired: 1 out]
          n206 = Equal?(x=w620, y=w621) -> (x = y?=w619:bool)
        }
        n207 = Search 1D Array(1D array=w609, element=TRUE) -> (index of element=w607:i32)  [unwired: 1 in]
        n208 = property on="Property Node" class="TabCtl (strict)"(reference=w608, error in=w602, "Value"=w607) -> (error out=w601:errorcluster)  [unwired: 1 out]
        n209 = flat-sequence "Log Line Builder" {
          tunnel: ["Set settings tab to: " ("String")] -> w616
          tunnel: [w623] -> w615
          tunnel: w601 -> [w624]
          tunnel: [w624] -> w614
          tunnel: w605 -> [w623]
          frame #0 {
          }
        }
      }
      event Panel Close? {
        w630 = TRUE  # Discard? T - Don't close panel.
        # "Shutdown and quit"
        n210 = event-data() -> ()  [unwired: 1 in, 4 out]
        n211 = event-data ("Event Filter Node")("Discard?"=w630) -> ()  [unwired: 1 in, 1 out]
      }
      event "Intensity Graph 2", "Intensity Graph": Scale Range Change {
        # "When intensity graph range changes resize pane objects (in order to keep correct aspect ratio)"
        n212 = event-data() -> ("CtlRef"=w638:refnum<vi>, "ScaleRef"=w635:refnum<vi>, "NewRange"=w634:T13)  [unwired: 1 in, 5 out]
        n213 = property on="Property Node" class="IntGraph (strict)"(reference=w638, error in=w633) -> (reference out=w636:refnum<vi>, error out=w632:errorcluster, "OwningPane"=w637:refnum<vi>)
        n214 = call-dynamic "ResizeObjectsinPane.vi"("error in (no error)"=w632, "PaneRef"=w637, "5PanesGUI in"=w641) -> ("error out"=w639:errorcluster, "5PanesGUI out"=w640:refnum<class "5PanesGUI.lvclass">)  [unwired: 7 in]
        n215 = flat-sequence "Log Line Builder" {
          tunnel: [w657] -> w644
          tunnel: ["" ("Empty String Constant")] -> w643
          tunnel: w639 -> [w647]
          tunnel: [w658] -> w642
          tunnel: w636 -> [w655]
          tunnel: w635 -> [w654]
          tunnel: w634 -> [w653]
          frame #0 {
            n216 = property on="Property Node" class="IntGraph (strict)"(reference=w655, error in=w647) -> (error out=w646:errorcluster, "Label.Text"=w652:string)  [unwired: 1 out]
            n217 = property on="Property Node" class="GrphScl"(reference=w654, error in=w646) -> (error out=w645:errorcluster, "NameLbl.Text"=w651:string)  [unwired: 1 out]
            n218 = Unbundle By Name(w653) -> ("Minimum"=w649:dbl, "Maximum"=w648:dbl)
            n219 = Format Into String(format string="Intensity graph \"%s\" axis %s range set: %f %f" ("decimal integer string"), error in=w645, w652, w651, w649, w648) -> (resulting string=w657:string, error out=w658:errorcluster)  [unwired: 1 in]
          }
        }
      }
      event Panel Resize {
        # "Front Panel resized"
        n220 = event-data() -> ()  [unwired: 1 in, 8 out]
        n221 = flat-sequence "Log Line Builder" {
          tunnel: [w671] -> w662
          tunnel: w661 -> [w670]
          tunnel: [w669] -> w660
          tunnel: ["FrontPanel resized: " ("String")] -> w659
          frame #0 {
            n222 = control-ref of="FP Bounds"() -> (w667:refnum<vi>)
            n223 = call "ClusterToDescriptiveString.vi"("error in"=w670, "Cluster In"=w667) -> ("error out"=w669:errorcluster, "String"=w671:string)  [unwired: 8 in]
          }
        }
        n224 = call "GetFPInfo.vi"("error in (no error)"=w664, "5PanesGUI in"=w666) -> ("error out"=w661:errorcluster, "Bounds"=→"FP Bounds":T9, "5PanesGUI out"=w665:refnum<class "5PanesGUI.lvclass">)  [unwired: 6 in, 1 out]
      }
      event "Developed By\nLEAP CODE\nLinking hardware \nwith software\n\nYoni Cohen": Mouse Down {
        # "Opens my linkedin profile in default browser when clicking on link"
        n225 = event-data() -> ("Button"=w672:u16)  [unwired: 1 in, 7 out]
        n226 = case shown="1" w672 {
          tunnel: [w678 w683] -> w676
          tunnel: [w679 "Open Linkedin page: " ("String")] -> w675
          tunnel: w674 -> [w678 w681]
          tunnel: [w679 w680] -> w673
          frame Default {
            w679 = "" ("String")
          }
          frame 1 {
            w680 = "https://www.linkedin.com/in/yoni-cohen-a03421110/"
            n227 = call-poly <vilib>:"Open URL in Default Browser.vi"("error in (no error)"=w681, "URL"=w680) -> ("error out"=w683:errorcluster)  [unwired: 4 in, 1 out]
          }
        }
      }
      event "Icon set by": Mouse Down {
        # "Opens icons8 website in default browser when clicking on link"
        n228 = event-data() -> ("CtlRef"=w689:refnum<vi>)  [unwired: 1 in, 7 out]
        n229 = property on="Property Node" class="Str"(reference=w689, error in=w685) -> (error out=w684:errorcluster, "Text.Text"=w686:string)  [unwired: 1 out]
        n230 = call-poly <vilib>:"Open URL in Default Browser.vi"("error in (no error)"=w684, "URL"=w686) -> ("error out"=w688:errorcluster)  [unwired: 4 in, 1 out]
      }
    }
    n231 = control-ref of="Listbox"() -> (w168:refnum<vi>)
    n232 = call "AddTextLineToListBox.vi"("error in (no error)"=w160, "String2"=w161, "String"=w169, "ListBox in"=w168) -> ("error out"=w159:errorcluster)  [unwired: 7 in]
    "Eventloop Error" <- w159
    n233 = call <vilib>:"Simple Error Handler.vi"("error in (no error)"=w159) -> ("error out"=w158:errorcluster)  [unwired: 4 in, 4 out]
  }
  n234 = call "ShutDown5Panes.vi"("error in (no error)"=w25, "5PanesGUI in"=w23) -> ("error out"=w22:errorcluster)  [unwired: 9 in]
  n235 = call <vilib>:"Simple Error Handler.vi"("error in (no error)"=w22) -> ()  [unwired: 4 in, 5 out]
  "Init Error" <- w5
